vi "Dummy Data SubVI.vi"(10 "Number of Columns":i32, 11 "Number of Rows":i32) -> (3 "Array":string[][](array[string]))   [LabVIEW 2015]
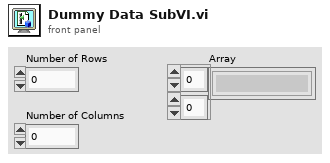
[diagram p1: front panel]
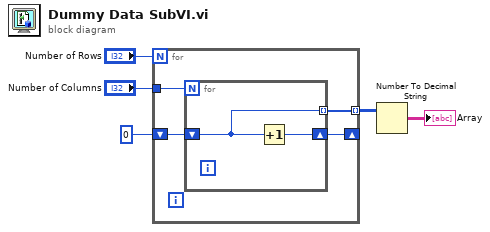
[diagram p0: block diagram]
diagram:
  n1 = for {
    N: "Number of Rows" -> [_]
    shift-right: [w8] -> _
    shift-left: 0 -> [w9]
    tunnel: [w7] -> w2 mode=indexing
    tunnel: "Number of Columns" -> [w6]
    n2 = for {
      N: w6 -> [_]
      shift-right: [w11] -> w8
      shift-left: w9 -> [w10]
      tunnel: [w10] -> w7 mode=indexing
      n3 = Increment(x=w10) -> (x+1=w11:i32)
    }
  }
  n4 = Number To Decimal String(number=w2) -> (decimal integer string=→"Array":string[][])  [unwired: 1 in]
